vi "ExecuteClimb.vi"(8 "Error In":errorcluster, 10 "Left Climb":T1={"DeviceStatus"={"status"=FALSE, "code"=0, "source"=""}, "Type"=enum."PWM", "PWM"={"PWM Channel"=enum."PWM 1", "DeadBand"={"Name"="", "maxPositivePwm"=0, "minPositivePwm"=0, "centerPwm"=0, "maxNegativePwm"=0, "minNegativePwm"=0, "angularRange"=0}}, "CAN"={"Device Number"=0, "SetOutput VI Ref"=variant(enum8{"Percent VBus", "Current", "Speed", "Position", "Voltage"} enum."Percent VBus"), "GetOutput VI Ref"=variant(refnum<k1> refnum), "Enable VI Ref"=variant(dbl 12.0), "Disable VI Ref"=variant(enum8{"Percent VBus", "Speed", "Position", "Slave", "Unchanged / Invalid", "Voltage Compensation", "Current", "Motion Profile"} enum."Percent VBus"), "Data"=variant}, "Invert"=FALSE, "DIO PWM"={"PWM \"Enable\" Channel"=enum."Invalid", "DIOChannel"=enum."Invalid", "PWM Rate"=0.0}}, 11 "Right Climb":T1={"DeviceStatus"={"status"=FALSE, "code"=0, "source"=""}, "Type"=enum."PWM", "PWM"={"PWM Channel"=enum."PWM 1", "DeadBand"={"Name"="", "maxPositivePwm"=0, "minPositivePwm"=0, "centerPwm"=0, "maxNegativePwm"=0, "minNegativePwm"=0, "angularRange"=0}}, "CAN"={"Device Number"=0, "SetOutput VI Ref"=variant(enum8{"Percent VBus", "Current", "Speed", "Position", "Voltage"} enum."Percent VBus"), "GetOutput VI Ref"=variant(refnum<k1> refnum), "Enable VI Ref"=variant(dbl 12.0), "Disable VI Ref"=variant(enum8{"Percent VBus", "Speed", "Position", "Slave", "Unchanged / Invalid", "Voltage Compensation", "Current", "Motion Profile"} enum."Percent VBus"), "Data"=variant}, "Invert"=FALSE, "DIO PWM"={"PWM \"Enable\" Channel"=enum."Invalid", "DIOChannel"=enum."Invalid", "PWM Rate"=0.0}}) -> (0 "Error Out":errorcluster)   [LabVIEW 2020]
uses:
  <vilib>/Rock Robotics/WPI/MotorControl/WPI_MotorControlDeviceRef.ctl
  <vilib>/Rock Robotics/WPI/MotorControl/WPI_MotorControlType.ctl
  <vilib>/Rock Robotics/SystemInterfaces/DIO/FPGA_DIOPWMChannel.ctl
  <vilib>/Rock Robotics/WPI/PWM/WPI_PWMDeadband.ctl
  <vilib>/Rock Robotics/SystemInterfaces/DIO/FPGA_DIOChannel.ctl
  <vilib>/Rock Robotics/WPI/ThirdParty/Phoenix-LabVIEW/Motor Controller/Controls/CTRE_Phoenix_MotorControl_ControlMode.ctl
  <vilib>/Rock Robotics/WPI/Solenoid/WPI_SolenoidValue.ctl
  ClimbGlobals.vi
  <vilib>/Rock Robotics/WPI/Solenoid/WPI_SolenoidSetEnum.vi
  <vilib>/Rock Robotics/WPI/ThirdParty/Phoenix-LabVIEW/Motor Controller/Get/CTRE_Phoenix_MotorController_GetLimitSwitchStates.vi
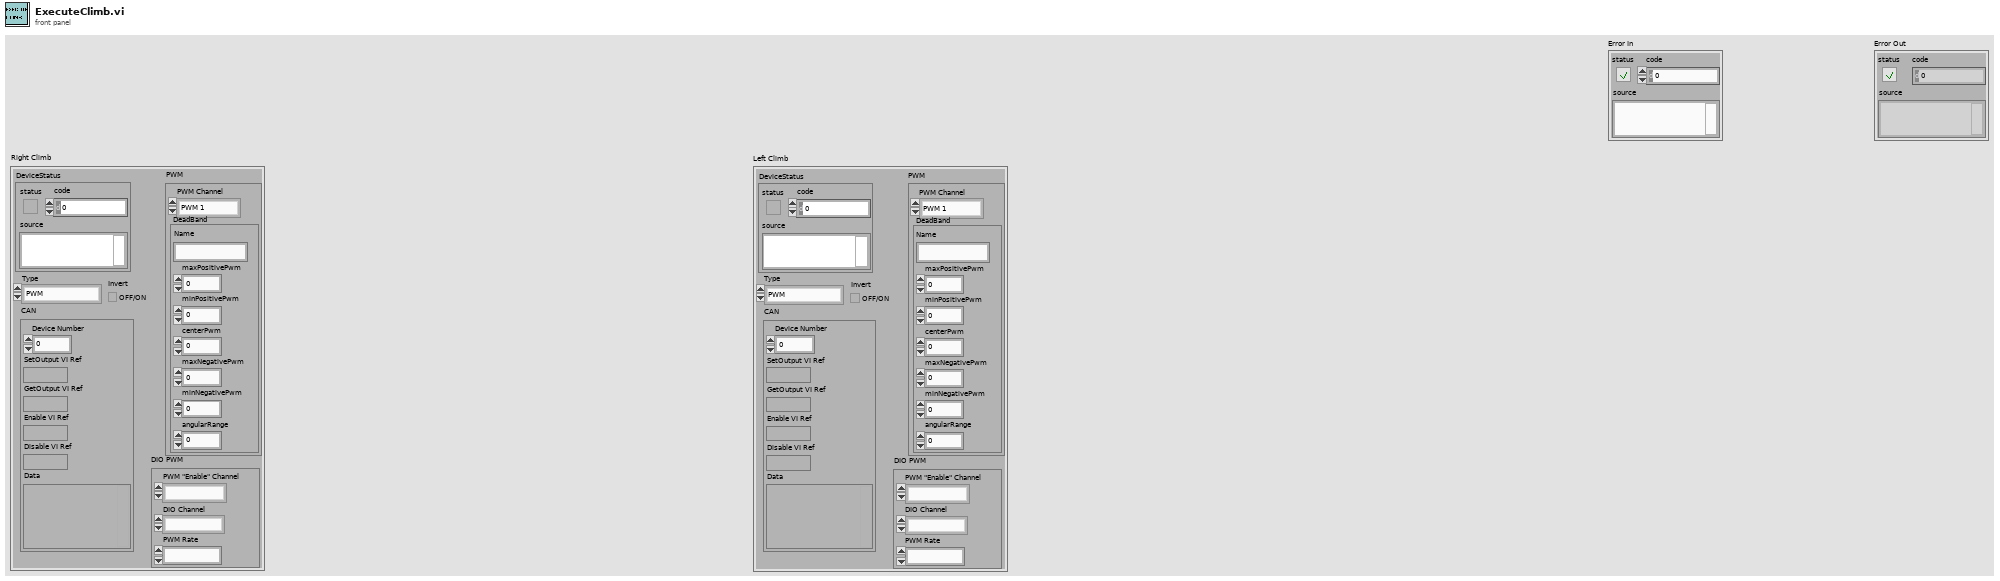
[diagram p1: front panel]
types:
  T1 = typedef "WPI_MotorControlDeviceRef.ctl" = cluster{"DeviceStatus":errorcluster, "Type":T2, "PWM":cluster{"PWM Channel":T3, "DeadBand":T4}, "CAN":cluster{"Device Number":u8, "SetOutput VI Ref":variant, "GetOutput VI Ref":variant, "Enable VI Ref":variant, "Disable VI Ref":variant, "Data":variant}, "Invert":bool, "DIO PWM":cluster{"PWM \"Enable\" Channel":T3, "DIOChannel":T5, "PWM Rate":dbl}}
  T2 = typedef "WPI_MotorControlType.ctl" = enum16{"PWM", "CAN", "DIO PWM"}
  T3 = typedef "FPGA_DIOPWMChannel.ctl" = enum8{"PWM 0", "PWM 1", "PWM 2", "PWM 3", "PWM 4", "PWM 5", "PWM 6", "PWM 7", "PWM 8", "PWM 9", "PWM MXP 0", "PWM MXP 1", "PWM MXP 2", "PWM MXP 3", "PWM MXP 4", "PWM MXP 5", "PWM MXP 6", "PWM MXP 7", "PWM MXP 8", "PWM MXP 9", "Invalid"}
  T4 = typedef "WPI_PWMDeadband.ctl" = cluster{"Name":string, "maxPositivePwm":i32, "minPositivePwm":i32, "centerPwm":i32, "maxNegativePwm":i32, "minNegativePwm":i32, "angularRange":u16}
  T5 = typedef "FPGA_DIOChannel.ctl" = enum8{"DIO 0", "DIO 1", "DIO 2", "DIO 3", "DIO 4", "DIO 5", "DIO 6", "DIO 7", "DIO 8", "DIO 9", "DIO MXP 0", "DIO MXP 1", "DIO MXP 2", "DIO MXP 3", "DIO MXP 4", "DIO MXP 5", "DIO MXP 6", "DIO MXP 7", "DIO MXP 8", "DIO MXP 9", "DIO MXP 10", "DIO MXP 11", "DIO MXP 12", "DIO MXP 13", "DIO MXP 14", "DIO MXP 15", "SPI Port CS1", "SPI Port CS2", "SPI Port CS3", "SPI Port MISO", "SPI Port MOSI", "Invalid"}
  T6 = typedef "WPI_SolenoidValue.ctl" = enum16{"Off", "On", "Forward", "Reverse"}
  T7 = typedef "CTRE_Phoenix_MotorControl_ControlMode.ctl" = u16
  T8 = typedef "WPI_SolenoidDevRef.ctl" = cluster{"DevStatus":errorcluster, "Pneumatics Control Module":u8, "Forward Solenoid Channel":T9, "Reverse Solenoid Channel":T9}
  T9 = typedef "WPI_SolenoidChannel.ctl" = enum8{"Solenoid 0", "Solenoid 1", "Solenoid 2", "Solenoid 3", "Solenoid 4", "Solenoid 5", "Solenoid 6", "Solenoid 7", "Solenoid 8", "Solenoid 9", "Solenoid 10", "Solenoid 11", "Solenoid 12", "Solenoid 13", "Solenoid 14", "Solenoid 15", "Invalid"}
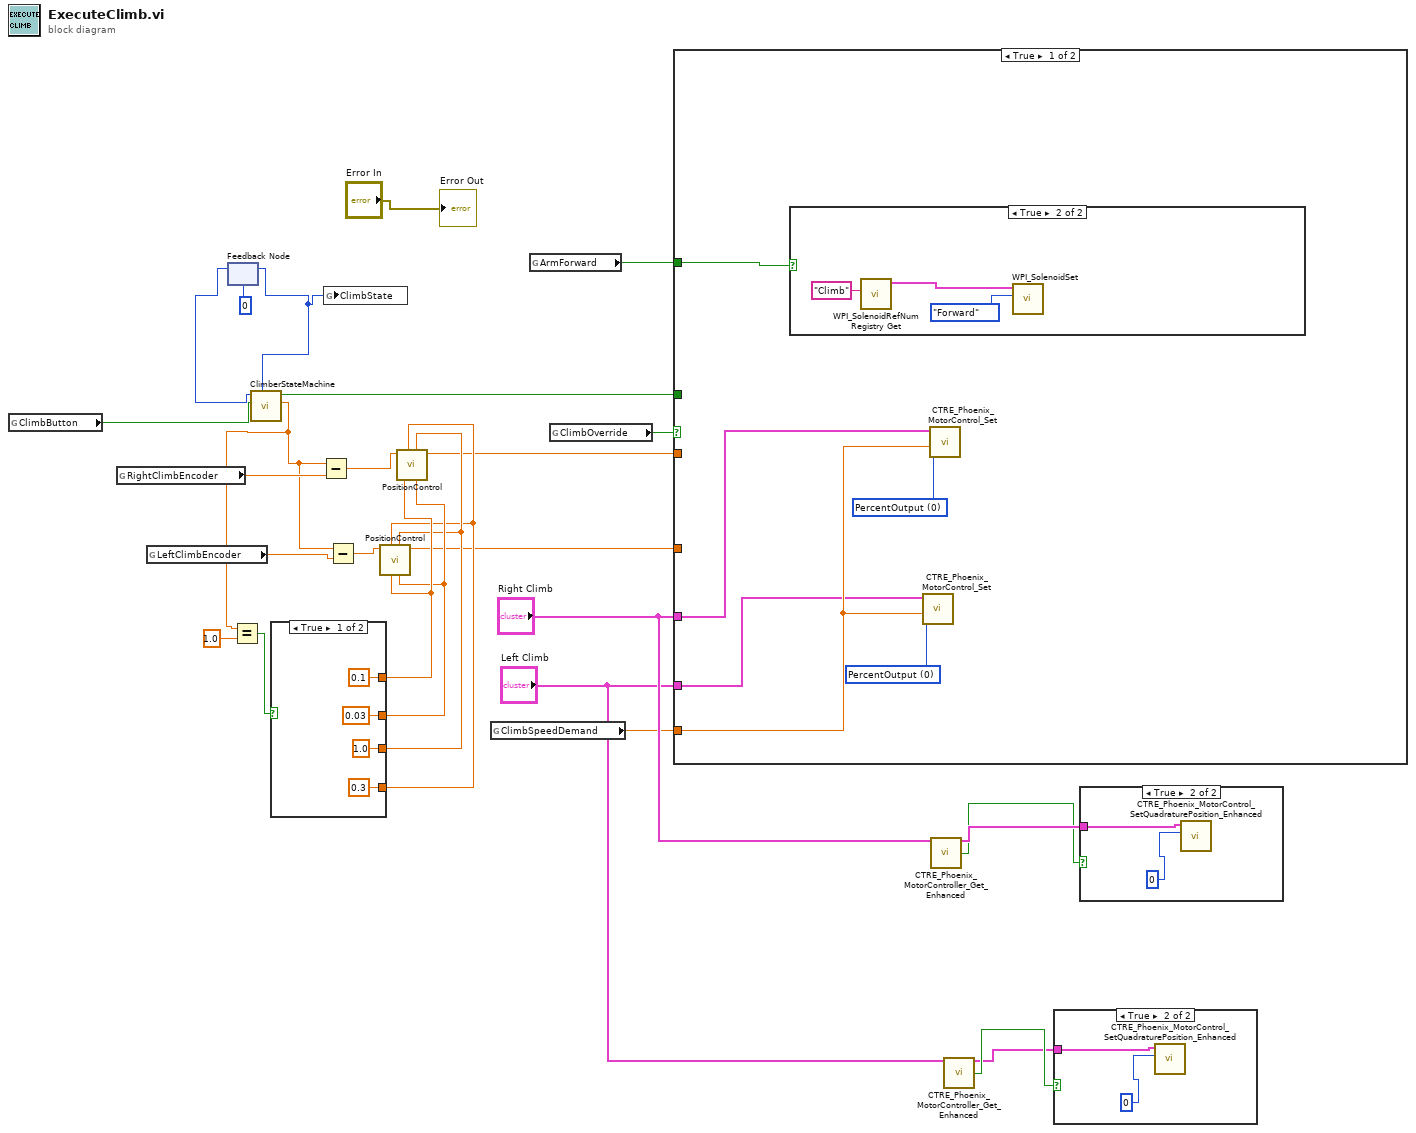
[diagram p0: block diagram]
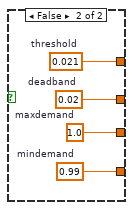
[diagram p4: hidden frame]
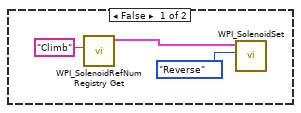
[diagram p5: hidden frame]
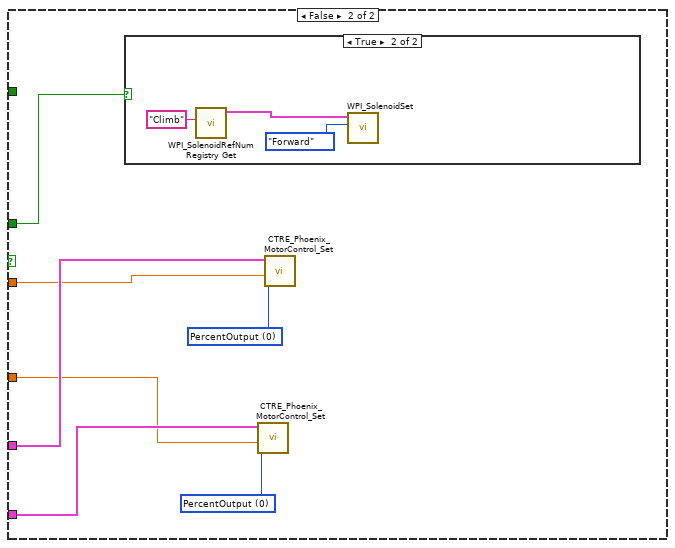
[diagram p6: hidden frame]
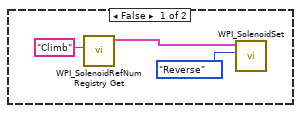
[diagram p7: hidden frame]
diagram:
  n1 = global read "ClimbGlobals.vi" "ClimbButton"() -> (w26:bool)
  n2 = global read "ClimbGlobals.vi" "RightClimbEncoder"() -> (w21:dbl)
  n3 = global read "ClimbGlobals.vi" "LeftClimbEncoder"() -> (w22:dbl)
  n4 = feedback #1(0 ("NextState")) -> (w28:i32)
  n5 = call "ClimberStateMachine.vi"("ClimbButton"=w26, "State"=w28) -> ("ArmPosition"=w8:dbl, "ArmForward"=w13:bool, "NextState"=w25:i32)  [unwired: 7 in]
  n6 = feedback-in #1(w25) -> ()
  n7 = Equal?(x=w8, y=1.0) -> (x = y?=w6:bool)
  n8 = case shown="True" w6 {
    tunnel: [0.1 ("threshold") w36] -> w18
    tunnel: [0.03 ("deadband") w35] -> w17
    tunnel: [1.0 ("maxdemand") w34] -> w16
    tunnel: [0.3 ("mindemand") w33] -> w15
    frame True {
    }
    frame False {
      w36 = 0.021  # threshold
      w35 = 0.02  # deadband
      w33 = 0.99  # mindemand
      w34 = 1.0  # maxdemand
    }
  }
  n9 = Subtract(x=w8, y=w21) -> (x-y=w20:dbl)
  n10 = global write "ClimbGlobals.vi" "ClimbState"(w25) -> ()
  n11 = Subtract(x=w8, y=w22) -> (x-y=w19:dbl)
  n12 = call "PositionControl.vi"("deadband"=w17, "maxdemand"=w16, "threshold"=w18, "mindemand"=w15, "Error"=w19) -> ("output variable"=w11:dbl)  [unwired: 5 in, 1 out]
  n13 = call "PositionControl.vi"("deadband"=w17, "maxdemand"=w16, "threshold"=w18, "mindemand"=w15, "Error"=w20) -> ("output variable"=w12:dbl)  [unwired: 5 in, 1 out]
  n14 = global read "ClimbGlobals.vi" "ClimbSpeedDemand"() -> (w14:dbl)
  n15 = global read "ClimbGlobals.vi" "ArmForward"() -> (w23:bool)
  n16 = global read "ClimbGlobals.vi" "ClimbOverride"() -> (w9:bool)
  n17 = case shown="True" w9 {
    tunnel: "Right Climb" -> [w38 w55]
    tunnel: "Left Climb" -> [w37 w53]
    tunnel: w23 -> [w40 _]
    tunnel: w14 -> [w39 _]
    tunnel: w13 -> [_ w51]
    tunnel: w12 -> [_ w50]
    tunnel: w11 -> [_ w49]
    frame True {
      w41 = T7 0 items=["PercentOutput"=0, "Position"=1, "Velocity"=2, "Current"=3, "Follower"=5, "MotionProfile"=6, "MotionMagic"=7, "MotionProfileArc"=10, "Disabled"=15] ("Control Mode")
      w42 = T7 0 items=["PercentOutput"=0, "Position"=1, "Velocity"=2, "Current"=3, "Follower"=5, "MotionProfile"=6, "MotionMagic"=7, "MotionProfileArc"=10, "Disabled"=15] ("Control Mode")
      n18 = case shown="True" w40 {
        frame False {
          n19 = call <vilib>:"WPI_SolenoidRefNum Registry Get.vi"("refnum name"="Climb") -> ("SolenoidDevRef"=w44:T8)  [unwired: 9 in, 1 out]
          n20 = call-poly <vilib>:"WPI_SolenoidSet.vi"("Value"=WPI_SolenoidValue."Reverse", "SolenoidDevRef"=w44) -> ()  [unwired: 8 in, 2 out]
        }
        frame True {
          n21 = call <vilib>:"WPI_SolenoidRefNum Registry Get.vi"("refnum name"="Climb") -> ("SolenoidDevRef"=w47:T8)  [unwired: 9 in, 1 out]
          n22 = call-poly <vilib>:"WPI_SolenoidSet.vi"("Value"=WPI_SolenoidValue."Forward", "SolenoidDevRef"=w47) -> ()  [unwired: 8 in, 2 out]
        }
      }
      n23 = call <vilib>:"CTRE_Phoenix_MotorControl_Set.vi"("Output"=w39, "Control Mode"=w41, "PhoenixMotorControlDevRef"=w37) -> ()  [unwired: 7 in, 2 out]
      n24 = call <vilib>:"CTRE_Phoenix_MotorControl_Set.vi"("Output"=w39, "Control Mode"=w42, "PhoenixMotorControlDevRef"=w38) -> ()  [unwired: 7 in, 2 out]
    }
    frame False {
      w52 = T7 0 items=["PercentOutput"=0, "Position"=1, "Velocity"=2, "Current"=3, "Follower"=5, "MotionProfile"=6, "MotionMagic"=7, "MotionProfileArc"=10, "Disabled"=15] ("Control Mode")
      w54 = T7 0 items=["PercentOutput"=0, "Position"=1, "Velocity"=2, "Current"=3, "Follower"=5, "MotionProfile"=6, "MotionMagic"=7, "MotionProfileArc"=10, "Disabled"=15] ("Control Mode")
      n25 = case shown="True" w51 {
        frame False {
          n26 = call <vilib>:"WPI_SolenoidRefNum Registry Get.vi"("refnum name"="Climb") -> ("SolenoidDevRef"=w57:T8)  [unwired: 9 in, 1 out]
          n27 = call-poly <vilib>:"WPI_SolenoidSet.vi"("Value"=WPI_SolenoidValue."Reverse", "SolenoidDevRef"=w57) -> ()  [unwired: 8 in, 2 out]
        }
        frame True {
          n28 = call <vilib>:"WPI_SolenoidRefNum Registry Get.vi"("refnum name"="Climb") -> ("SolenoidDevRef"=w60:T8)  [unwired: 9 in, 1 out]
          n29 = call-poly <vilib>:"WPI_SolenoidSet.vi"("Value"=WPI_SolenoidValue."Forward", "SolenoidDevRef"=w60) -> ()  [unwired: 8 in, 2 out]
        }
      }
      n30 = call <vilib>:"CTRE_Phoenix_MotorControl_Set.vi"("Output"=w49, "Control Mode"=w52, "PhoenixMotorControlDevRef"=w53) -> ()  [unwired: 7 in, 2 out]
      n31 = call <vilib>:"CTRE_Phoenix_MotorControl_Set.vi"("Output"=w50, "Control Mode"=w54, "PhoenixMotorControlDevRef"=w55) -> ()  [unwired: 7 in, 2 out]
    }
  }
  n32 = call-poly <vilib>:"CTRE_Phoenix_MotorController_Get_Enhanced.vi"("PhoenixMotorControlDevRef"="Right Climb") -> ("PhoenixMotorControlDevRef"=w4:T1, "Reverse Limit Closed?"=w2:bool)  [unwired: 11 in, 2 out]
  n33 = call-poly <vilib>:"CTRE_Phoenix_MotorController_Get_Enhanced.vi"("PhoenixMotorControlDevRef"="Left Climb") -> ("PhoenixMotorControlDevRef"=w1:T1, "Reverse Limit Closed?"=w3:bool)  [unwired: 11 in, 2 out]
  n34 = case shown="True" w3 {
    tunnel: w1 -> [_ w63]
    frame False {
    }
    frame True {
      n35 = call <vilib>:"CTRE_Phoenix_MotorControl_SetQuadraturePosition_Enhanced.vi"("New Position"=0, "PhoenixMotorControlDevRef"=w63) -> ()  [unwired: 8 in, 2 out]
    }
  }
  n36 = case shown="True" w2 {
    tunnel: w4 -> [_ w65]
    frame False {
    }
    frame True {
      n37 = call <vilib>:"CTRE_Phoenix_MotorControl_SetQuadraturePosition_Enhanced.vi"("New Position"=0, "PhoenixMotorControlDevRef"=w65) -> ()  [unwired: 8 in, 2 out]
    }
  }
  "Error Out" <- "Error In"
